vi "Structures-Labelled.vi"   [LabVIEW 2019]
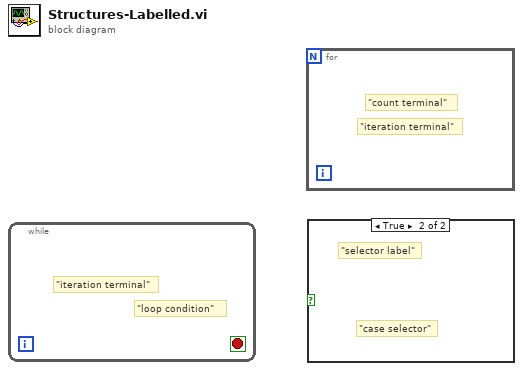
[diagram p0: block diagram]
diagram:
  n1 = while {
    stop <- _ stop-if-true
    # "\"iteration terminal\""
    # "\"loop condition\""
  }
  n2 = for {
    # "\"count terminal\""
    # "\"iteration terminal\""
  }
  n3 = case shown="True" {
    selector: _ -> [_ _]
    frame False {
    }
    frame True {
      # "\"selector label\""
      # "\"case selector\""
    }
  }
